vi "LVClass_ModalCoef GetLegendrePrefs.vi"(0 "ModalCoef in":refnum<class "ModalCoef.lvclass">, 11 "error in (no error)":errorcluster) -> (4 "ModalCoef out":refnum<class "ModalCoef.lvclass">, 6 "LegendreModalPrefs":T1={"Number of coefficients"=32, "Filtered coefficients"=[], "RMS Legendre normalization"=FALSE, "RectangularProjectionPupilDimensions"={"Pupil center_sspp"={"X"=0.0, "Y"=0.0}, "Pupil halfsize_sspp"={"X"=0.0, "Y"=0.0}}}, 15 "error out":errorcluster)   [LabVIEW 2020, in "ModalCoef.lvclass"]
doc: "Get preferences for phase reconstruction from Legendre decomposition.\n\n--------------------------------------------------------------------------------\n\n<B>ComputePhaseSetIn </B> : ComputePhaseSet object.\n<B>ComputePhaseSetOut </B> : ComputePhaseSet object.\n<B>nb_coeffs_total </B> : Number of the Legendre coefficients used in the polynomial base.\n<B>nb_coeffs_to_filter </B> : Number of the Legendre coefficients to filter in the polynomial base.\n<B>coeffs_to_filter </B> : Indices of the Legendre coefficients to filter in the polynomial base.\n<B>projection_pupil_center </B> : Center of the projection pupil,in number of subpupils.\n<B>projection_pupil_halfsize </B> : Projection pupil half-size, in number of subpupils.\n<B>ErrorIn </B> : Error\n<B>ErrorOut </B> : Error\n\n--------------------------------------------------------------------------------"
uses:
  ModalCoef.lvclass
  LegendreModalPrefs.ctl
  LegendreProjectionPupilSetup.ctl
  Point2Df.ctl
  ModalCoef.lvclass/ModalCoef.ctl
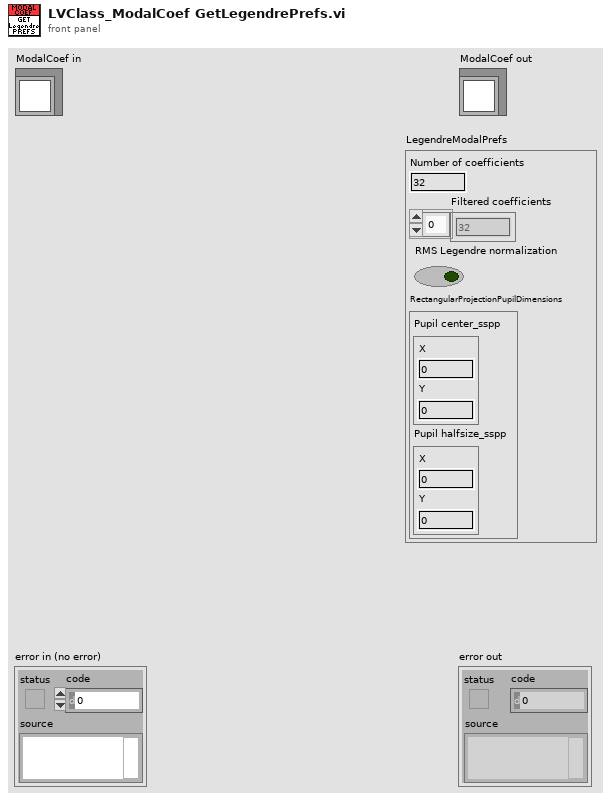
[diagram p1: front panel]
types:
  T1 = typedef "LegendreModalPrefs.ctl" = cluster{"Number of coefficients":u32, "Filtered coefficients":u32[], "RMS Legendre normalization":bool, "RectangularProjectionPupilDimensions":T2}
  T2 = typedef "LegendreProjectionPupilSetup.ctl" = cluster{"Pupil center_sspp":T3, "Pupil halfsize_sspp":T3}
  T3 = typedef "Point2Df.ctl" = cluster{"X":sgl, "Y":sgl}
  T4 = typedef "ClassID.ctl" = i64
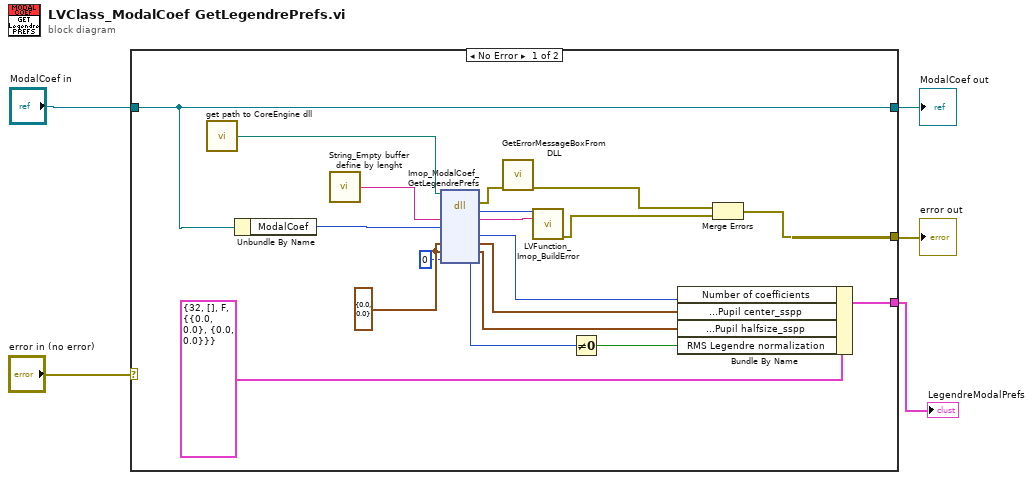
[diagram p0: block diagram]
diagram:
  n1 = case shown="No Error" "error in (no error)" {
    selector: "error in (no error)" -> [_ w26]
    tunnel: [w10 w26] -> w2
    tunnel: [w14 w25] -> w4
    tunnel: "ModalCoef in" -> [w14 w25]
    tunnel: [w19 _] -> w1
    frame No Error {
      w17 = T3 {"X"=0.0, "Y"=0.0} ("RectangularProjectionPupilDimensions.Pupil center_sspp")
      n2 = call "get path to CoreEngine dll.vi"() -> ("path to wavekit library"=w21:path)  [unwired: 14 in, 1 out]
      n3 = Unbundle By Name(w14) -> ("ModalCoef"=w13:T4)
      n4 = call "String_Empty buffer define by lenght.vi"() -> ("Empty buffer"=w22:string)  [unwired: 1 in]
      n5 = dll-call lib="D:/2_trunk/Soft_haso/ImOpCoreEngine4_LV2011/DLLs/ImopEngine4_vc100.dll" fn="Imop_ModalCoef_GetLegendrePrefs"(path in=w21, "message"=w22, "objet"=w13, "projection_pupil_center"=w17, "projection_pupil_size"=w17, "normalization"=u8 0) -> (error out=w20:errorcluster, "return type"=w24:i32, "message"=w23:string, "numberOfCoefficient"=w15:u32, "projection_pupil_center"=w18:T3, "projection_pupil_size"=w16:T3, "normalization"=w9:u8)  [unwired: 4 in, 1 out]
      n6 = call "GetErrorMessageBoxFromDLL.vi"("error IN"=w20) -> ("error OUT"=w12:errorcluster)  [unwired: 10 in]
      n7 = call "LVFunction_Imop_BuildError.vi"("code"=w24, "String to Prepend to source (\"\")"=w23) -> ("error out"=w11:errorcluster)  [unwired: 13 in]
      n8 = Not Equal To 0?(x=w9) -> (x != 0?=w6:bool)
      n9 = Bundle By Name(cluster=T1 {"Number of coefficients"=32, "Filtered coefficients"=[], "RMS Legendre normalization"=FALSE, "RectangularProjectionPupilDimensions"={"Pupil center_sspp"={"X"=0.0, "Y"=0.0}, "Pupil halfsize_sspp"={"X"=0.0, "Y"=0.0}}} ("LegendreModalPrefs"), "Number of coefficients"=w15, "RectangularProjectionPupilDimensions.Pupil center_sspp"=w18, "RectangularProjectionPupilDimensions.Pupil halfsize_sspp"=w16, "RMS Legendre normalization"=w6) -> (w19:T1)
      n10 = Merge Errors(w12, w11) -> (w10:errorcluster)
    }
    frame Error {
    }
  }
  "error out" <- w2
  "ModalCoef out" <- w4
  "LegendreModalPrefs" <- w1
